vi "Capacitance Parameters.vi"(0 "Data Management Control":T1, 2 "Specific Voltages":dbl[](array[numeric])=[32.0, 36.0], 5 "Selected Exp Settings":T2={"P2_Sweep_Stop_V"=36.0, "P2_Sweep_Step_V"=1.0, "Experiment Name"="", "Resistance Threshold"=1.0, "P1_Fixed_Voltage"=36.0, "P2_Sweep_Start_V"=36.0}, 11 "Error In":errorcluster, 13 "Cal Measurements":T3 {"Port 3 Capacitance" format="%#_6p"; "Port 2 Capacitance" format="%#_6p"; "Port 1 Capacitance" format="%#_6p"}) -> (4 "Capacitance Calculated Values":T4, 6 "Cap Calc Arrays":T5={"CPD_sum"=[], "P2_CPD@V"=[], "P1_CPD@V"=[], "Specific Voltages"=[32.0, 36.0]}, 8 "Corrected_Capacitance Calculated Values":T6, 15 "Error Out":errorcluster)   [LabVIEW 2013]
uses:
  Controls/Data Management.ctl
  Controls/Individual User Inputs.ctl
  Controls/Capacitance Individual Calculated Values.ctl
  Controls/Capacitance Array Calculated Values.ctl
  Controls/ENA_Marker Measurements.ctl
  Controls/Corrected_Capacitance Individual Calculated Values.ctl
panel:
  in  "Tab Control":enum32{"Inputs", "Outputs"}(tab)
  # "Test Settings"
  # "Make the Stop and Step Negative \nfor negative sweep"
  # "Calculation Settings"
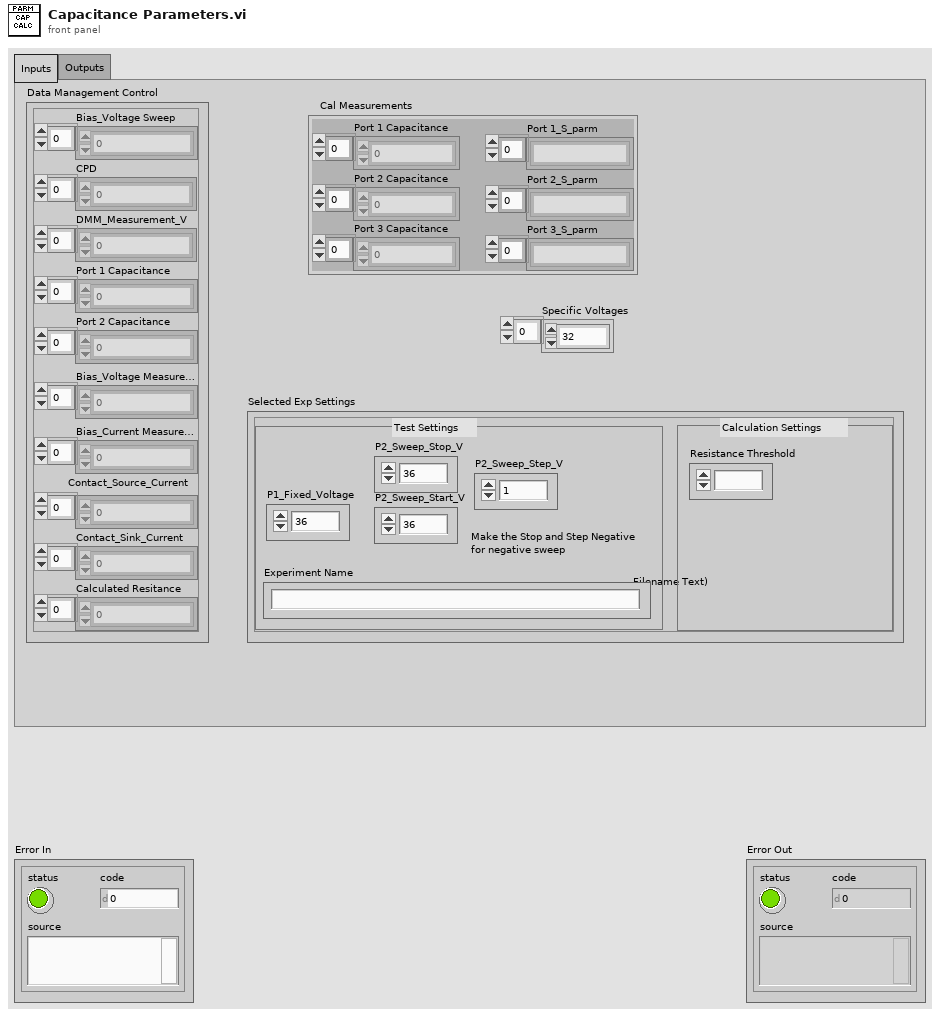
[diagram p1: front panel]
types:
  T1 = typedef "Data Management.ctl" = cluster{"Bias_Voltage Sweep":dbl[], "CPD":dbl[], "DMM_Measurement_V":dbl[], "Port 1 Capacitance":dbl[], "Port 2 Capacitance":dbl[], "Bias_Voltage Measurement":dbl[], "Bias_Current Measurement":dbl[], "Contact_Source_Current":dbl[], "Contact_Sink_Current":dbl[], "Calculated Resitance":dbl[]}
  T2 = typedef "Individual User Inputs.ctl" = cluster{"P2_Sweep_Stop_V":dbl, "P2_Sweep_Step_V":dbl, "Experiment Name":string, "Resistance Threshold":dbl, "P1_Fixed_Voltage":dbl, "P2_Sweep_Start_V":dbl}
  T3 = typedef "ENA_Marker Measurements.ctl" = cluster{"Port 1 Capacitance":dbl[], "Port 2 Capacitance":dbl[], "Port 3 Capacitance":dbl[], "Port 1_S_parm":string[], "Port 2_S_parm":string[], "Port 3_S_parm":string[]}
  T4 = typedef "Capacitance Individual Calculated Values.ctl" = cluster{"P1_CPD_free":dbl, "P2_CPD_free":dbl, "P1_CPD_vmax":dbl, "P2_CPD_vmax":dbl, "P1_CPD_first":dbl, "P2_CPD_first":dbl, "P1_CPD_last":dbl, "P2_CPD_last":dbl, "P1_CPD_end":dbl, "P2_CPD_end":dbl, "P1_CPD_max":dbl, "P2_CPD_max ":dbl, "CPD_Free":dbl, "CPD_First":dbl, "CPD_max":dbl, "CPD_Last":dbl, "CPD_End":dbl, "CPD_vmax":dbl}
  T5 = typedef "Capacitance Array Calculated Values.ctl" = cluster{"CPD_sum":dbl[], "P2_CPD@V":dbl[], "P1_CPD@V":dbl[], "Specific Voltages":dbl[]}
  T6 = typedef "Corrected_Capacitance Individual Calculated Values.ctl" = cluster{"P1_CPD_free":dbl, "P2_CPD_free":dbl, "P1_CPD_vmax":dbl, "P2_CPD_vmax":dbl, "P1_CPD_first":dbl, "P2_CPD_first":dbl, "P1_CPD_last":dbl, "P2_CPD_last":dbl, "P1_CPD_end":dbl, "P2_CPD_end":dbl, "P1_CPD_max":dbl, "P2_CPD_max ":dbl, "CPD_Free":dbl, "CPD_First":dbl, "CPD_max":dbl, "CPD_Last":dbl, "CPD_End":dbl, "CPD_vmax":dbl}
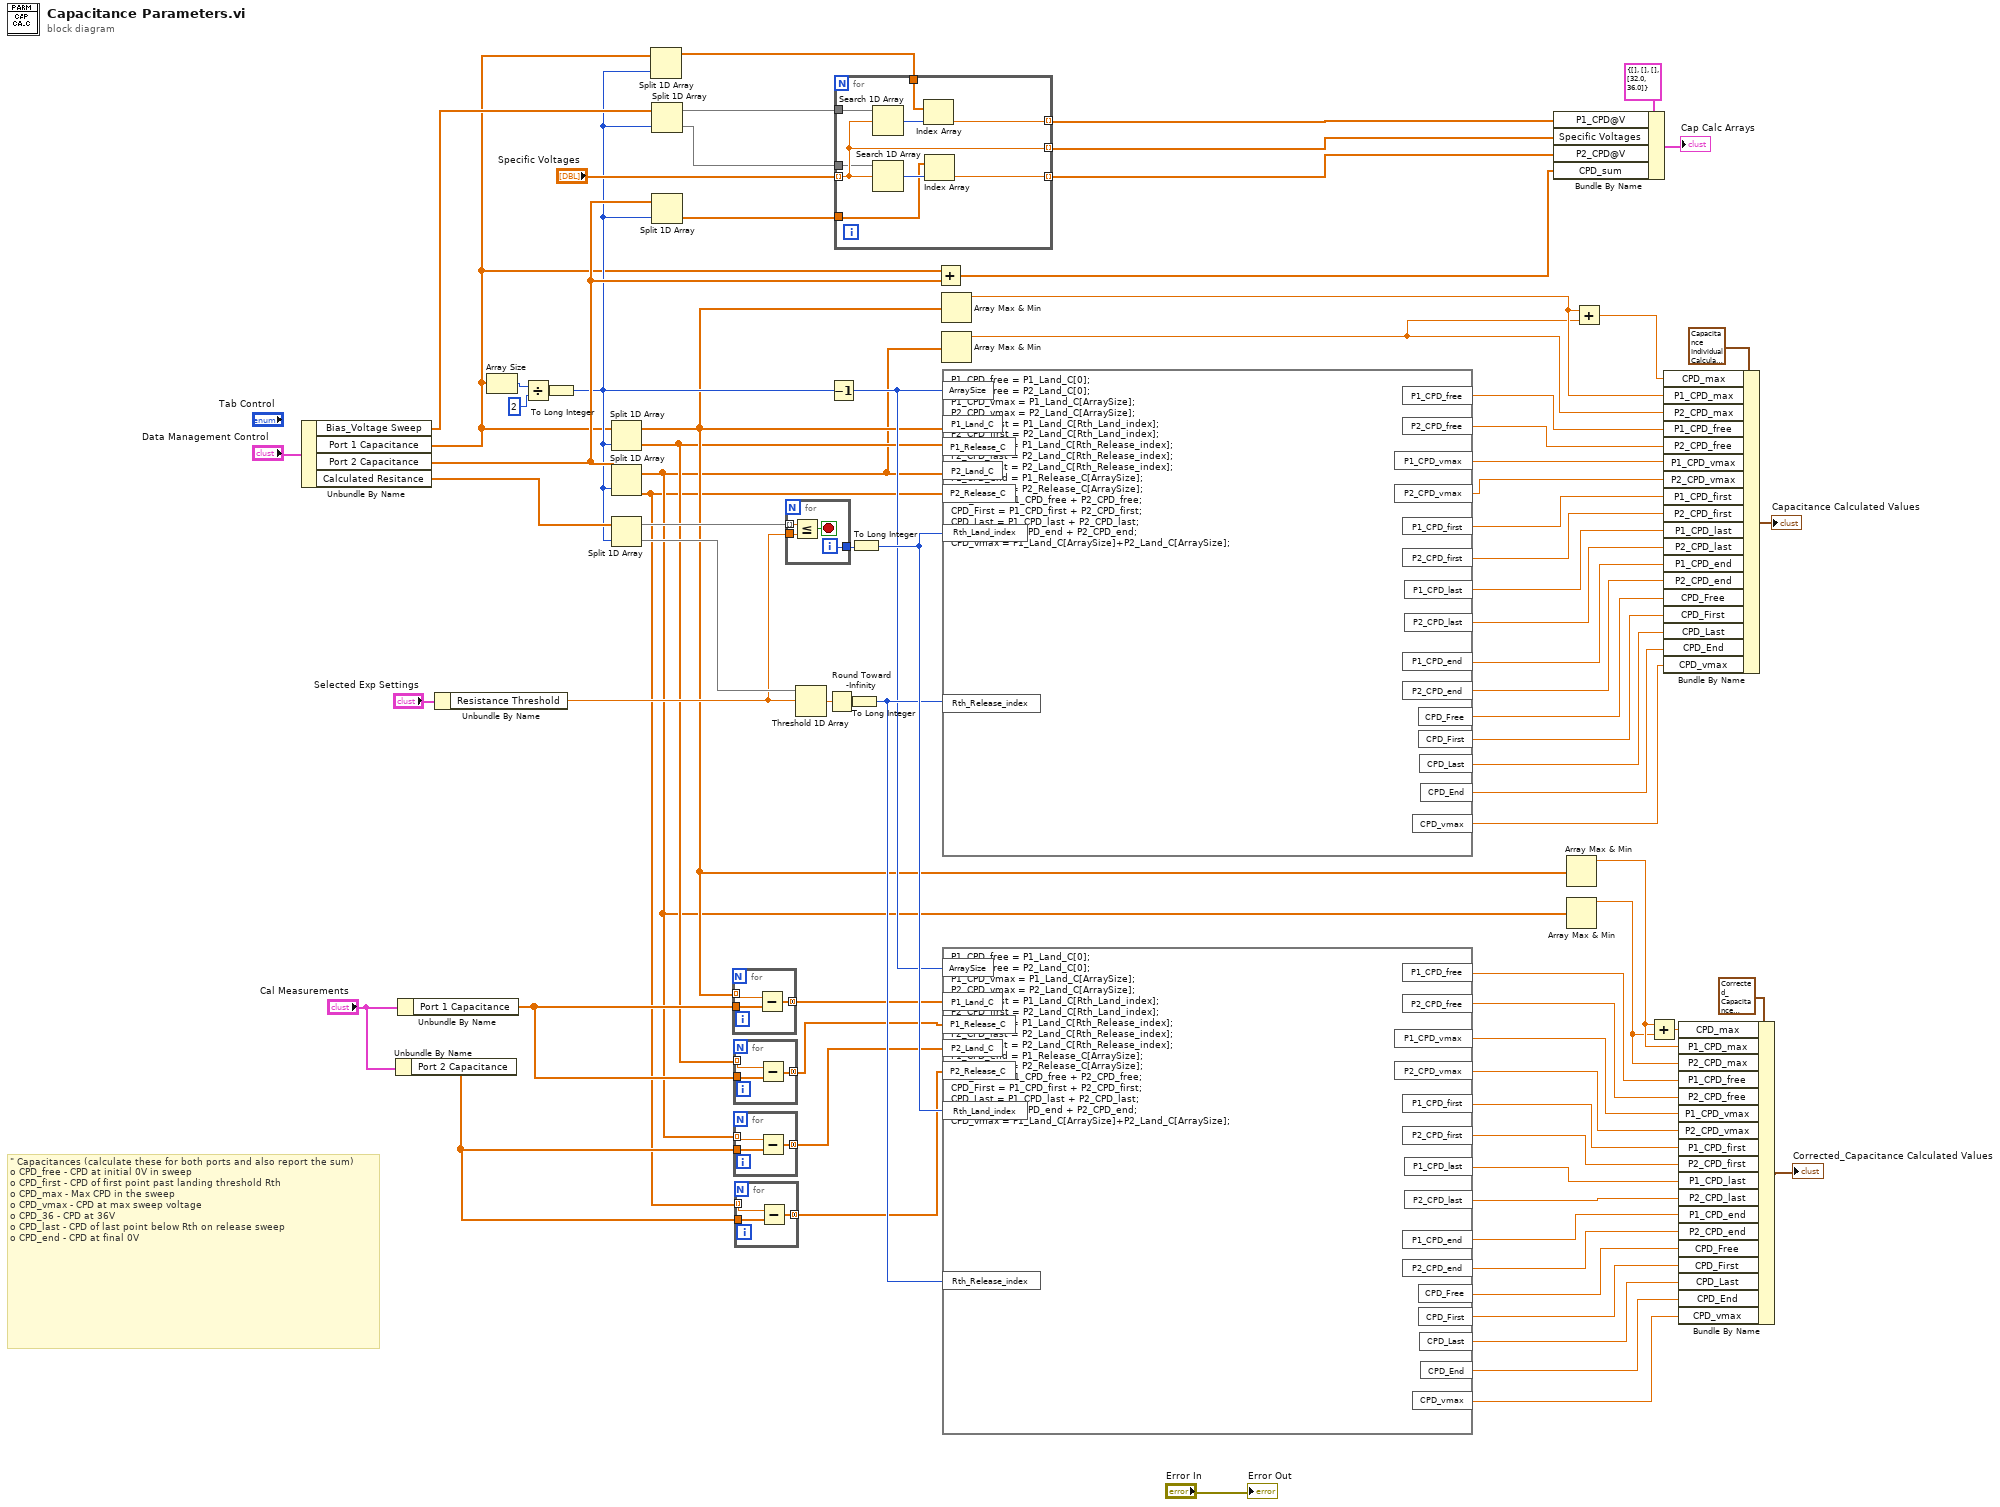
[diagram p0: block diagram]
diagram:
  # "\"\tCapacitances (calculate these for both ports and also report the sum)\no\tCPD_free - CPD at initial 0V in sweep\no\tCPD_first - CPD of first point past landing threshold Rth \no\tCPD_max - Max CPD in the sweep\no\tCPD_vmax - CPD at max sweep voltage\no\tCPD_36 - CPD at 36V\no\tCPD_last - CPD of last point below Rth on release sweep\no\tCPD_end - CPD at final 0V"
  n1 = Unbundle By Name("Data Management Control") -> ("Bias_Voltage Sweep"=w74:dbl[], "Port 1 Capacitance"=w12:dbl[], "Port 2 Capacitance"=w73:dbl[], "Calculated Resitance"=w78:dbl[])
  n2 = Unbundle By Name("Cal Measurements") -> ("Port 2 Capacitance"=w5:dbl[])
  n3 = Unbundle By Name("Cal Measurements") -> ("Port 1 Capacitance"=w9:dbl[])
  n4 = Unbundle By Name("Selected Exp Settings") -> ("Resistance Threshold"=w38:dbl)
  n5 = Array Size(array=w12) -> (size(s)=w81:i32)
  n6 = Divide(x=w81, y=2) -> (x/y=w79:dbl)
  n7 = To Long Integer(number=w79) -> (32bit integer=w59:i32)
  n8 = Split 1D Array(array=w12, index=w59) -> (first subarray=w11:dbl[], second subarray=w8:dbl[])
  n9 = Split 1D Array(array=w73, index=w59) -> (first subarray=w6:dbl[], second subarray=w2:dbl[])
  n10 = Split 1D Array(array=w78, index=w59) -> (first subarray=w39:dbl[], second subarray=w77:dbl[])
  n11 = Split 1D Array(array=w12, index=w59) -> (first subarray=w57:dbl[])  [unwired: 1 out]
  n12 = Split 1D Array(array=w74, index=w59) -> (first subarray=w55:dbl[], second subarray=w54:dbl[])
  n13 = Split 1D Array(array=w73, index=w59) -> (second subarray=w72:dbl[])  [unwired: 1 out]
  n14 = for {
    tunnel: w9 -> [w85]
    tunnel: [w84] -> w10 mode=concatenating
    tunnel: w11 -> [w83] mode=indexing
    n15 = Subtract(x=w83, y=w85) -> (x-y=w84:dbl[])
  }
  n16 = for {
    tunnel: w9 -> [w88]
    tunnel: [w87] -> w7 mode=concatenating
    tunnel: w8 -> [w86] mode=indexing
    n17 = Subtract(x=w86, y=w88) -> (x-y=w87:dbl[])
  }
  n18 = for {
    tunnel: w5 -> [w91]
    tunnel: [w90] -> w3 mode=concatenating
    tunnel: w6 -> [w89] mode=indexing
    n19 = Subtract(x=w89, y=w91) -> (x-y=w90:dbl[])
  }
  n20 = for {
    tunnel: w5 -> [w94]
    tunnel: [w93] -> w1 mode=concatenating
    tunnel: w2 -> [w92] mode=indexing
    n21 = Subtract(x=w92, y=w94) -> (x-y=w93:dbl[])
  }
  n22 = for {
    tunnel: [w98] -> w37
    tunnel: w39 -> [w96] mode=indexing
    tunnel: w38 -> [w95]
    i -> [w98]
    stop <- w97 stop-if-true
    n23 = Less Or Equal?(x=w96, y=w95) -> (x <= y?=w97:bool)
  }
  n24 = Threshold 1D Array(2:w38, 3:w77) -> (0:w76:dbl)  [unwired: 1 in]
  n25 = Round Toward -Infinity(1:w76) -> (0:w75:dbl)
  n26 = Decrement(x=w59) -> (x-1=w15:i32)
  n27 = for {
    tunnel: "Specific Voltages" -> [w105] mode=indexing
    tunnel: [w106] -> w49 mode=indexing
    tunnel: [w105] -> w50 mode=indexing
    tunnel: w55 -> [w104]
    tunnel: w54 -> [w102]
    tunnel: w57 -> [w101]
    tunnel: [w100] -> w51 mode=indexing
    tunnel: w72 -> [w99]
    n28 = Search 1D Array(1D array=w104, element=w105) -> (index of element=w103:i32)  [unwired: 1 in]
    n29 = Search 1D Array(1D array=w102, element=w105) -> (index of element=w107:i32)  [unwired: 1 in]
    n30 = Index Array(array=w101, index=w103) -> (element=w100:dbl)
    n31 = Index Array(array=w99, index=w107) -> (element=w106:dbl)
  }
  n32 = To Long Integer(number=w75) -> (32bit integer=w34:i32)
  n33 = To Long Integer(number=w37) -> (32bit integer=w35:i32)
  n34 = Add(x=w12, y=w73) -> (x+y=w48:dbl[])
  n35 = Array Max & Min(array=w11) -> (max value=w46:dbl)  [unwired: 3 out]
  n36 = Array Max & Min(array=w6) -> (max value=w45:dbl)  [unwired: 3 out]
  n37 = formula code="P1_CPD_free = P1_Land_C[0];\nP2_CPD_free = P2_Land_C[0];\nP1_CPD_vmax = P1_Land_C[ArraySize];\nP2_CPD_vmax = P2_Land_C[ArraySize];\nP1_CPD_first = P1_Land_C[Rth_Land_index];\nP2_CPD_first = P2_Land_C[Rth_Land_index];\nP1_CPD_last = P1_Land_C[Rth_Release_index];\nP2_CPD_last = P2_Land_C[Rth_Release_index];\nP2_CPD_last = P2_Land_C[Rth_Release_index];\nP1_CPD_end = P1_Release_C[ArraySize];\nP2_CPD_end = P2_Release_C[ArraySize];\nCPD_Free = P1_CPD_free + P2_CPD_free;\nCPD_First = P1_CPD_first + P2_CPD_first;\nCPD_Last = P1_CPD_last + P2_CPD_last;\nCPD_End = P1_CPD_end + P2_CPD_end;\nCPD_vmax = P1_Land_C[ArraySize]+P2_Land_C[ArraySize];"("P1_Land_C"=w11, "P2_Land_C"=w6, "ArraySize"=w15, "Rth_Land_index"=w35, "Rth_Release_index"=w34, "P1_Release_C"=w8, "P2_Release_C"=w2) -> ("P1_CPD_free"=w56:dbl, "P2_CPD_free"=w69:dbl, "P1_CPD_vmax"=w68:dbl, "P2_CPD_vmax"=w67:dbl, "P1_CPD_first"=w66:dbl, "P2_CPD_first"=w65:dbl, "P1_CPD_last"=w64:dbl, "P2_CPD_last"=w63:dbl, "P1_CPD_end"=w62:dbl, "P2_CPD_end"=w61:dbl, "CPD_Free"=w43:dbl, "CPD_First"=w42:dbl, "CPD_Last"=w41:dbl, "CPD_End"=w40:dbl, "CPD_vmax"=w36:dbl)
  n38 = formula code="P1_CPD_free = P1_Land_C[0];\nP2_CPD_free = P2_Land_C[0];\nP1_CPD_vmax = P1_Land_C[ArraySize];\nP2_CPD_vmax = P2_Land_C[ArraySize];\nP1_CPD_first = P1_Land_C[Rth_Land_index];\nP2_CPD_first = P2_Land_C[Rth_Land_index];\nP1_CPD_last = P1_Land_C[Rth_Release_index];\nP2_CPD_last = P2_Land_C[Rth_Release_index];\nP2_CPD_last = P2_Land_C[Rth_Release_index];\nP1_CPD_end = P1_Release_C[ArraySize];\nP2_CPD_end = P2_Release_C[ArraySize];\nCPD_Free = P1_CPD_free + P2_CPD_free;\nCPD_First = P1_CPD_first + P2_CPD_first;\nCPD_Last = P1_CPD_last + P2_CPD_last;\nCPD_End = P1_CPD_end + P2_CPD_end;\nCPD_vmax = P1_Land_C[ArraySize]+P2_Land_C[ArraySize];"("P1_Land_C"=w10, "P2_Land_C"=w3, "ArraySize"=w15, "Rth_Land_index"=w35, "Rth_Release_index"=w34, "P1_Release_C"=w7, "P2_Release_C"=w1) -> ("P1_CPD_free"=w30:dbl, "P2_CPD_free"=w29:dbl, "P1_CPD_vmax"=w28:dbl, "P2_CPD_vmax"=w27:dbl, "P1_CPD_first"=w26:dbl, "P2_CPD_first"=w25:dbl, "P1_CPD_last"=w24:dbl, "P2_CPD_last"=w23:dbl, "P1_CPD_end"=w22:dbl, "P2_CPD_end"=w21:dbl, "CPD_Free"=w20:dbl, "CPD_First"=w19:dbl, "CPD_Last"=w18:dbl, "CPD_End"=w17:dbl, "CPD_vmax"=w16:dbl)
  n39 = Bundle By Name(cluster=T5 {"CPD_sum"=[], "P2_CPD@V"=[], "P1_CPD@V"=[], "Specific Voltages"=[32.0, 36.0]} ("Cap Calc Arrays 2"), "P1_CPD@V"=w51, "Specific Voltages"=w50, "P2_CPD@V"=w49, "CPD_sum"=w48) -> (→"Cap Calc Arrays":T5)
  n40 = Array Max & Min(array=w11) -> (max value=w32:dbl)  [unwired: 3 out]
  n41 = Array Max & Min(array=w6) -> (max value=w31:dbl)  [unwired: 3 out]
  n42 = Add(x=w46, y=w45) -> (x+y=w44:dbl)
  n43 = Add(x=w32, y=w31) -> (x+y=w33:dbl)
  n44 = Bundle By Name(cluster=T4 {"P1_CPD_free"=0.0, "P2_CPD_free"=0.0, "P1_CPD_vmax"=0.0, "P2_CPD_vmax"=0.0, "P1_CPD_first"=0.0, "P2_CPD_first"=0.0, "P1_CPD_last"=0.0, "P2_CPD_last"=0.0, "P1_CPD_end"=0.0, "P2_CPD_end"=0.0, "P1_CPD_max"=0.0, "P2_CPD_max "=0.0, "CPD_Free"=0.0, "CPD_First"=0.0, "CPD_max"=0.0, "CPD_Last"=0.0, "CPD_End"=0.0, "CPD_vmax"=0.0} ("Capacitance Calculated Values"), "CPD_max"=w44, "P1_CPD_max"=w46, "P2_CPD_max"=w45, "P1_CPD_free"=w56, "P2_CPD_free"=w69, "P1_CPD_vmax"=w68, "P2_CPD_vmax"=w67, "P1_CPD_first"=w66, "P2_CPD_first"=w65, "P1_CPD_last"=w64, "P2_CPD_last"=w63, "P1_CPD_end"=w62, "P2_CPD_end"=w61, "CPD_Free"=w43, "CPD_First"=w42, "CPD_Last"=w41, "CPD_End"=w40, "CPD_vmax"=w36) -> (→"Capacitance Calculated Values":T4)
  n45 = Bundle By Name(cluster=T6 {"P1_CPD_free"=0.0, "P2_CPD_free"=0.0, "P1_CPD_vmax"=0.0, "P2_CPD_vmax"=0.0, "P1_CPD_first"=0.0, "P2_CPD_first"=0.0, "P1_CPD_last"=0.0, "P2_CPD_last"=0.0, "P1_CPD_end"=0.0, "P2_CPD_end"=0.0, "P1_CPD_max"=0.0, "P2_CPD_max "=0.0, "CPD_Free"=0.0, "CPD_First"=0.0, "CPD_max"=0.0, "CPD_Last"=0.0, "CPD_End"=0.0, "CPD_vmax"=0.0} ("Corrected_Capacitance Calculated Values"), "CPD_max"=w33, "P1_CPD_max"=w32, "P2_CPD_max"=w31, "P1_CPD_free"=w30, "P2_CPD_free"=w29, "P1_CPD_vmax"=w28, "P2_CPD_vmax"=w27, "P1_CPD_first"=w26, "P2_CPD_first"=w25, "P1_CPD_last"=w24, "P2_CPD_last"=w23, "P1_CPD_end"=w22, "P2_CPD_end"=w21, "CPD_Free"=w20, "CPD_First"=w19, "CPD_Last"=w18, "CPD_End"=w17, "CPD_vmax"=w16) -> (→"Corrected_Capacitance Calculated Values":T6)
  "Error Out" <- "Error In"
